vi "Set_TempUnit.vi"(0 "VisaCluster":T2, 7 "Temp_Unit":T1, 11 "error in (no error)":errorcluster) -> (4 "VisaCluster":T2, 6 "Temp_Unit":T1, 8 "Answer":string, 15 "error out":errorcluster)   [LabVIEW 2014, in "FH 55.lvlib"]
doc: "The VI selects one of three instrument operating modes: \nTemperature display off \nTemperature unit Celsius\nTemperature unit Fahrenheit.\n\nDurch das VI kann zwischen den folgenden Ausgaben gewählt werden:\nKeine Ausgabe auf dem Display,\nTemperatureinheit Celsius,\nTemperatureinheit Fahrenheit."
uses:
  FH 55.lvlib
  TypeDef/VisaCluster.ctl
  TypeDef/Temp_Unit.ctl
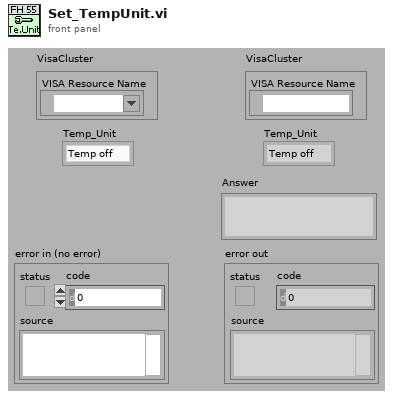
[diagram p1: front panel]
types:
  T1 = typedef "FH 55.lvlib/Temp_Unit.ctl" = enum16{"Temp off", "Celsius", "Fahrenheit"}
  T2 = typedef "FH 55.lvlib/VisaCluster.ctl" = cluster{"VISA Resource Name":refnum<visa-resource-name>}
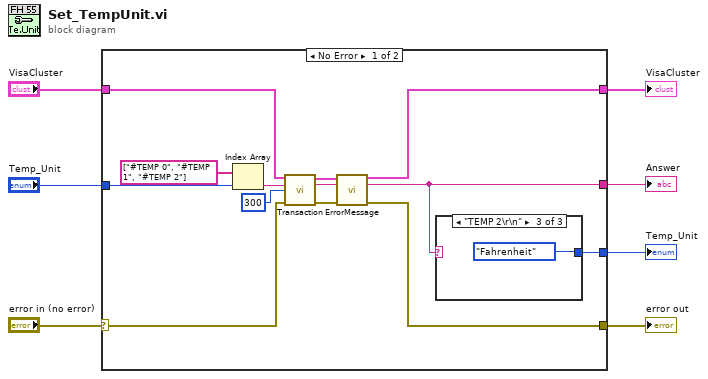
[diagram p0: block diagram]
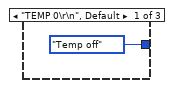
[diagram p2: hidden frame]
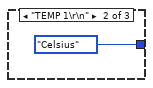
[diagram p3: hidden frame]
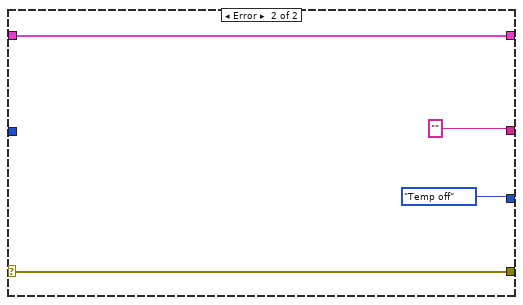
[diagram p4: hidden frame]
diagram:
  n1 = case shown="No Error" "error in (no error)" {
    selector: "error in (no error)" -> [w17 w26]
    tunnel: "VisaCluster" -> [w18 w27]
    tunnel: "Temp_Unit" -> [w13 _]
    tunnel: [w20 w27] -> w3
    tunnel: [w19 w26] -> w5
    tunnel: [w10 ""] -> w4
    tunnel: [w9 Temp_Unit."Temp off" ("Temp_Unit")] -> w1
    frame No Error {
      n2 = Index Array(array=string[] ["#TEMP 0", "#TEMP 1", "#TEMP 2"], index=w13) -> (element=w12:string)
      n3 = call "Transaction.vi"("VisaCluster"=w18, "Command"=w12, "Time (150) ms"=u32 300, "error in (no error)"=w17) -> ("VisaCluster"=w14:T2, "Answer"=w15:string, "error out"=w16:errorcluster)  [unwired: 8 in, 1 out]
      n4 = call "ErrorMessage.vi"("VisaCluster"=w14, "Message In"=w15, "error in (no error)"=w16) -> ("VisaCluster"=w20:T2, "Message Out"=w10:string, "error out"=w19:errorcluster)  [unwired: 10 in]
      n5 = case shown="\"TEMP 2\\r\\n\"" w10 {
        tunnel: [Temp_Unit."Temp off" ("Temp_Unit") Temp_Unit."Celsius" ("Temp_Unit") Temp_Unit."Fahrenheit" ("Temp_Unit")] -> w9
        frame "TEMP 0\r\n", Default {
        }
        frame "TEMP 1\r\n" {
        }
        frame "TEMP 2\r\n" {
        }
      }
    }
    frame Error {
    }
  }
  "error out" <- w5
  "Answer" <- w4
  "VisaCluster" <- w3
  "Temp_Unit" <- w1
